vi "Read DAQ Parameters.vi"(8 "error in (no error)":errorcluster, 11 "ATS9462 Class in":refnum<class "ATS9462 Class.lvclass">) -> (0 "error out":errorcluster, 2 "DAQ Parameters":T1, 3 "ATS9462 Class out":refnum<class "ATS9462 Class.lvclass">)   [LabVIEW 2015, in "ATS9462 Class.lvclass"]
uses:
  ATS9462 Class.lvclass
  DAQ Parameters.ctl
  Trigger Source.ctl
  Trigger Slope.ctl
  Type Defs/OCT DAQ Channel Data Type.ctl
  Clock Control.ctl
  DAQ Class.lvclass
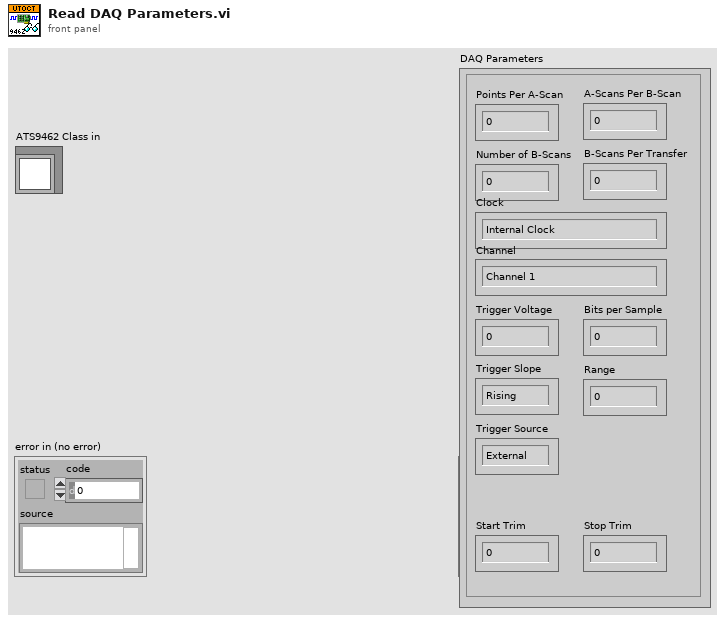
[diagram p1: front panel]
types:
  T1 = typedef "DAQ Class.lvclass/DAQ Parameters.ctl" = cluster{"Points Per A-Scan":u32, "A-Scans Per B-Scan":u32, "Number of B-Scans":u32, "B-Scans Per Transfer":u32, "Trigger Voltage":sgl, "Trigger Source":T2, "Trigger Slope":T3, "Channel":T4, "Clock":T5, "Bits per Sample":dbl, "Range":dbl, "Start Trim":u32, "Stop Trim":u32}
  T2 = typedef "DAQ Class.lvclass/Trigger Source.ctl" = enum16{"External", "Channel A", "Channel B"}
  T3 = typedef "DAQ Class.lvclass/Trigger Slope.ctl" = enum16{"Rising", "Falling"}
  T4 = typedef "OCT DAQ Channel Data Type.ctl" = enum16{"Channel 1", "Channel 2", "Channel 1 and 2"}
  T5 = typedef "DAQ Class.lvclass/Clock Control.ctl" = enum16{"Internal Clock", "External Clock"}
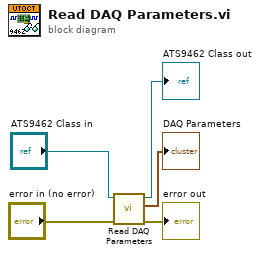
[diagram p0: block diagram]
diagram:
  n1 = call-parent "Read DAQ Parameters.vi"("error in (no error)"="error in (no error)", "DAQ Class in"="ATS9462 Class in") -> ("error out"=→"error out":errorcluster, "DAQ Parameters"=→"DAQ Parameters":T1, "DAQ Class out"=→"ATS9462 Class out":refnum<class "ATS9462 Class.lvclass">)  [unwired: 7 in]
